vi "Withdraw.vi"(8 "error in":errorcluster, 10 "Amount":string, 11 "PIN":string) -> (0 "error out":errorcluster, 2 "Tokens":cluster{"Name":string, "Amount":string}[](array[cluster]), 3 "Message":string)   [LabVIEW 2020]
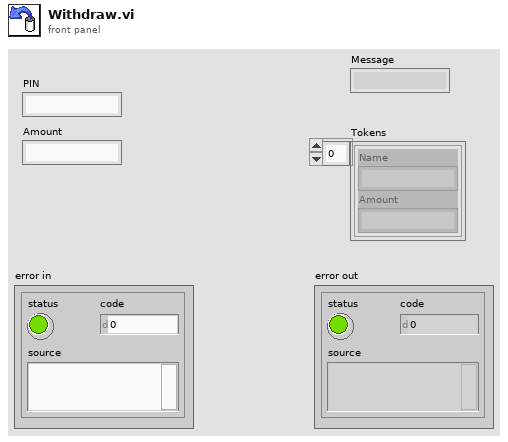
[diagram p1: front panel]
types:
  T1 = enum16{"Init", "Get Balance", "Update Balance", "Find Name"}
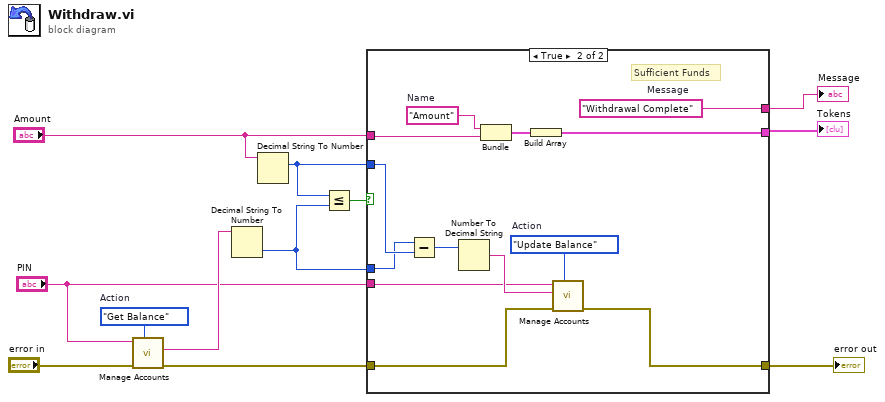
[diagram p0: block diagram]
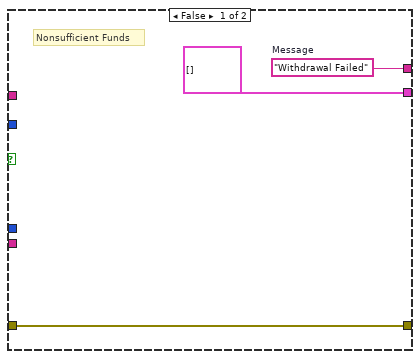
[diagram p2: hidden frame]
diagram:
  w12 = T1."Get Balance"  # Action
  n1 = call "Manage Accounts.vi"("Action"=w12, "error in (no error)"="error in", "PIN"="PIN") -> ("error out"=w7:errorcluster, "Get Value"=w11:string)  [unwired: 7 in]
  n2 = Decimal String To Number(string=w11) -> (number=w10:i32)  [unwired: 2 in, 1 out]
  n3 = Decimal String To Number(string="Amount") -> (number=w9:i32)  [unwired: 2 in, 1 out]
  n4 = Less Or Equal?(x=w9, y=w10) -> (x <= y?=w8:bool)
  n5 = case shown="True" w8 {
    tunnel: w10 -> [_ w22]
    tunnel: w9 -> [_ w23]
    tunnel: w7 -> [w14 w21]
    tunnel: [w14 w20] -> w2
    tunnel: [w13 w19] -> w4
    tunnel: "Amount" -> [_ w18]
    tunnel: [cluster{string, "User Input":string}[] [] w17] -> w5
    tunnel: "PIN" -> [_ w16]
    frame False {
      w13 = "Withdrawal Failed"  # Message
      # "Nonsufficient Funds"
    }
    frame True {
      w25 = "Amount"  # Name
      w19 = "Withdrawal Complete"  # Message
      w28 = T1."Update Balance"  # Action
      # "Sufficient Funds"
      n6 = Subtract(x=w22, y=w23) -> (x-y=w27:i32)
      n7 = Number To Decimal String(number=w27) -> (decimal integer string=w26:string)  [unwired: 1 in]
      n8 = Bundle("Name"=w25, "Amount"=w18) -> (w24:cluster{"Name":string, "Amount":string})  [unwired: 1 in]
      n9 = Build Array(w24) -> (w17:cluster{"Name":string, "Amount":string}[])
      n10 = call "Manage Accounts.vi"("Action"=w28, "error in (no error)"=w21, "Set Value"=w26, "PIN"=w16) -> ("error out"=w20:errorcluster)  [unwired: 6 in, 1 out]
    }
  }
  "error out" <- w2
  "Tokens" <- w5
  "Message" <- w4
